vi "while_v0_v19.vi"() -> ()   [LabVIEW 2009]
panel:
  in  "x1,y1":cluster{"x":i16, "y":i16}={"x"=355, "y"=257}
  in  "x0, y0":cluster{"x":i16, "y":i16}={"x"=50, "y"=70}
  in  "Culoarea":u32(colorbox)=16711695
  in  "stop":bool
  out "Picture":picture
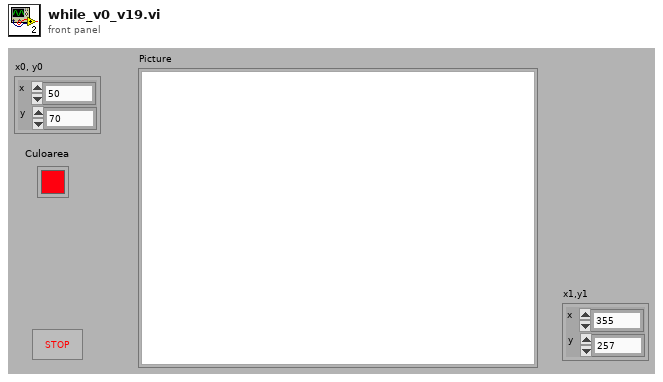
[diagram p1: front panel]
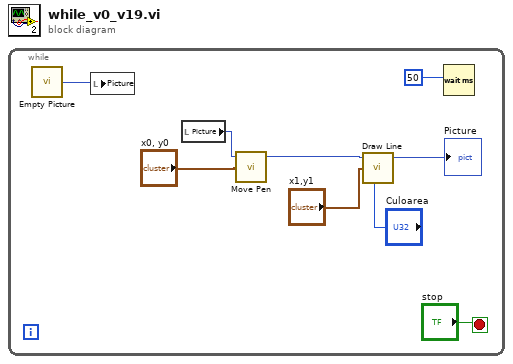
[diagram p0: block diagram]
diagram:
  n1 = while {
    stop <- "stop" stop-if-true
    n2 = call "Empty Picture"() -> ("empty picture"=w4:picture)
    n3 = local write "Picture"(w4) -> ()
    n4 = local read "Picture"() -> (w7:picture)
    n5 = call <vilib>:"Move Pen.vi"("new position"="x0, y0", "picture"=w7) -> ("new picture"=w6:picture)  [unwired: 3 in]
    n6 = call <vilib>:"Draw Line.vi"("picture"=w6, "end point"="x1,y1", "color(black)"="Culoarea") -> ("new picture"=→"Picture":picture)  [unwired: 6 in]
    n7 = Wait (ms)(milliseconds to wait=50) -> ()  [unwired: 1 out]
  }
